vi "Major.vi"(9 "c":u32 format="0x%08x", 10 "b":u32 format="0x%08x", 11 "a":u32 format="0x%08x") -> (2 "Major":u32 format="0x%08x")   [LabVIEW 2018, in "Crypto.lvlib" / "SHA-256.lvclass"]
uses:
  SHA-256.lvclass
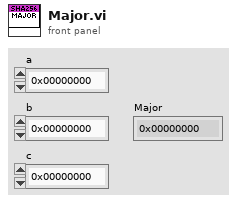
[diagram p1: front panel]
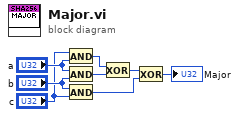
[diagram p0: block diagram]
diagram:
  n1 = And(x="c", y="a") -> (x .and. y?=w4:u32)
  n2 = And(x="a", y="b") -> (x .and. y?=w5:u32)
  n3 = And(x="b", y="c") -> (x .and. y?=w2:u32)
  n4 = Exclusive Or(1:w5, 2:w4) -> (0:w3:u32)
  n5 = Exclusive Or(1:w2, 2:w3) -> (0:→"Major":u32)
